vi "Restore Setup.vi"(8 "error in (no error)":errorcluster, 9 "Restore Setup File Location":path, 10 "Saved Setup Number (0)":i32, 11 "VISA resource name":refnum<visa-resource-name>) -> (0 "error out":errorcluster, 3 "VISA resource name out":refnum<visa-resource-name>)   [LabVIEW 2014, in "Fluke 190 Series II.lvlib"]
doc: "Restores a complete setup."
uses:
  Fluke 190 Series II.lvlib
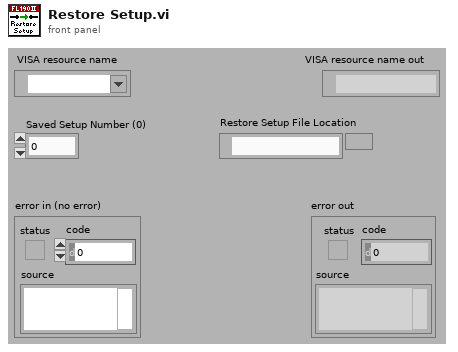
[diagram p1: front panel]
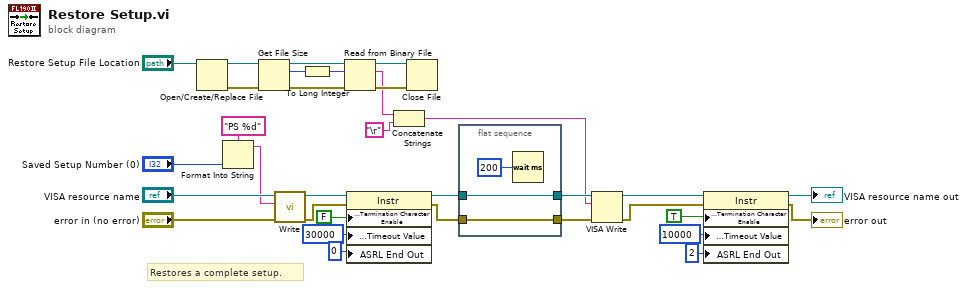
[diagram p0: block diagram]
diagram:
  # "Restores a complete setup."
  n1 = Open/Create/Replace File(file path (use dialog)="Restore Setup File Location") -> (refnum out=w15:refnum<file>, error out=w16:errorcluster)  [unwired: 5 in, 1 out]
  n2 = Format Into String(format string="PS %d", "Saved Setup Number (0)") -> (resulting string=w27:string)  [unwired: 2 in, 1 out]
  n3 = Get File Size(file=w15, error in=w16) -> (refnum out=w14:refnum<file>, size (in bytes)=w12:i64, 0:w13:errorcluster)
  n4 = call "Write.vi"("error in (no error)"="error in (no error)", "Write Buffer"=w27, "VISA resource name"="VISA resource name") -> ("error out"=w25:errorcluster, "VISA resource name out"=w26:refnum<visa-resource-name>)  [unwired: 7 out]
  n5 = To Long Integer(number=w12) -> (32bit integer=w11:i32)
  n6 = Read from Binary File(8:w13, 10:w11, 11:w14) -> (0:w10:errorcluster, 2:w8:string, 3:w9:refnum<file>)  [unwired: 4 out]
  n7 = property on="Property Node" class="Instr"(reference=w26, error in=w25, "Message Based Settings:Termination Character Enable"=FALSE, "General Settings:Timeout Value"=u32 30000, "ASRL End Out"=u16 0 ("Serial Settings:End Mode for Reads")) -> (reference out=w7:refnum<visa-resource-name>, error out=w6:errorcluster)
  n8 = Concatenate Strings(w8, "\r" ("Carriage Return Constant")) -> (w1:string)
  n9 = Close File(refnum=w9, error in=w10) -> ()  [unwired: 2 out]
  n10 = flat-sequence {
    tunnel: [w36] -> w5
    tunnel: w7 -> [w36]
    tunnel: w6 -> [w35]
    tunnel: [w35] -> w4
    frame #0 {
      n11 = Wait (ms)(milliseconds to wait=u32 200) -> ()  [unwired: 1 out]
    }
  }
  n12 = VISA Write(VISA resource name=w5, write buffer=w1, error in (no error)=w4) -> (VISA resource name out=w3:refnum<visa-resource-name>, error out=w2:errorcluster)  [unwired: 1 out]
  n13 = property on="Property Node" class="Instr"(reference=w3, error in=w2, "Message Based Settings:Termination Character Enable"=TRUE, "General Settings:Timeout Value"=u32 10000, "ASRL End Out"=u16 2 ("Serial Settings:End Mode for Reads")) -> (reference out=→"VISA resource name out":refnum<visa-resource-name>, error out=→"error out":errorcluster)
